vi "Check Start Button.vi"(8 "error in":errorcluster, 10 "Trigger Status":bool, 11 "Status Byte":u16) -> (0 "error out":errorcluster, 2 "Trigger Pressed?":bool)   [LabVIEW 2015, in "Tool Module.lvlib"]
uses:
  Tool Module.lvlib
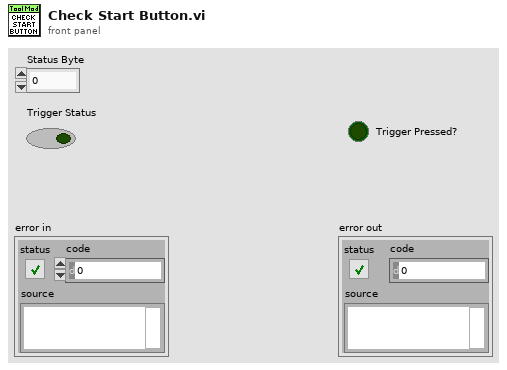
[diagram p1: front panel]
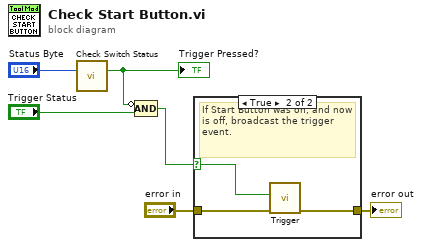
[diagram p0: block diagram]
diagram:
  n1 = call "Check Switch Status.vi"("Status Byte"="Status Byte") -> ("Trigger Pressed?"=w5:bool)  [unwired: 14 in]
  "Trigger Pressed?" <- w5
  n2 = Compound Arithmetic op=AND(invert w5, "Trigger Status") -> (w3:bool)
  n3 = case shown="True" w3 {
    selector: w3 -> [_ w10]
    tunnel: "error in" -> [w7 w9]
    tunnel: [w7 w8] -> w1
    frame False {
    }
    frame True {
      # "If Start Button was on, and now is off, broadcast the trigger event."
      n4 = call "Trigger.vi"("error in (no error)"=w9, "Trigger"=w10) -> ("error out"=w8:errorcluster)  [unwired: 9 in]
    }
  }
  "error out" <- w1
